vi "Elapsed Time.vi"() -> (3 "elapsed time (s)":dbl)   [LabVIEW 2019, in "Pet Feeder.lvlib"]
uses:
  Pet Feeder.lvlib
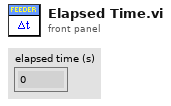
[diagram p1: front panel]
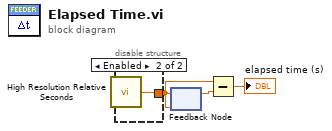
[diagram p0: block diagram]
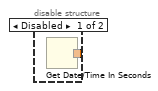
[diagram p2: hidden frame]
diagram:
  n1 = disable-structure shown="Enabled" {
    disable-tunnel: [w4 w5] -> w3
    frame Disabled {
      n2 = Get Date/Time In Seconds() -> (seconds since 1Jan1904=w4:timestamp)
    }
    frame Enabled {
      n3 = call <vilib>:"High Resolution Relative Seconds.vi"() -> ("relative seconds"=w5:dbl)
    }
  }
  n4 = feedback #1(w3) -> (w1:dbl)
  n5 = feedback-in #1(w3) -> ()
  n6 = Subtract(x=w3, y=w1) -> (x-y=→"elapsed time (s)":dbl)
